vi "Destroy Session.vi"(8 "error in (no error)":errorcluster, 11 "Session Handle":refnum<data-value>) -> (0 "error out":errorcluster)   [LabVIEW 2020, in "G-Embedded-Python-Interpreter-Toolkit.lvlib"]
uses:
  G-Embedded-Python-Interpreter-Toolkit.lvlib
  bin/gepit.cp310.32.dll
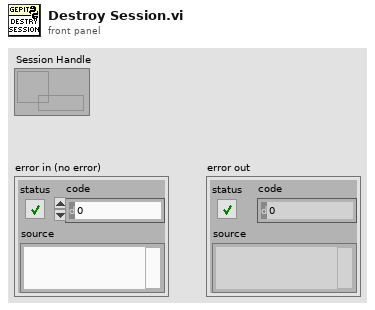
[diagram p1: front panel]
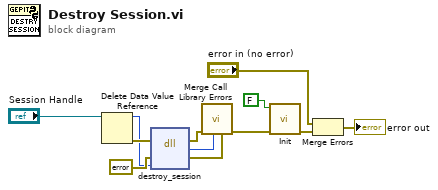
[diagram p0: block diagram]
diagram:
  n1 = Delete Data Value Reference(data value reference="Session Handle") -> (data value=w6:u64, error out=w7:errorcluster)  [unwired: 1 in]
  n2 = dll-call lib="C:/serenial/libraries/g-embedded-python-interpreter-toolkit/LabVIEW/bin/gepit.cp310.32.dll" fn="destroy_session"(error in=w7, "Error"=errorcluster {"status"=FALSE, "code"=0, "source"=""} ("error constant"), "Session"=w6) -> (error out=w11:errorcluster, "return type"=w10:i32, "Error"=w9:errorcluster)  [unwired: 3 in, 1 out]
  n3 = call "Merge Call Library Errors.vi"("Call Library Error"=w9, "Return Value"=w10, "error in"=w11) -> ("error out"=w3:errorcluster)  [unwired: 8 in]
  n4 = call "Init.vi"("error in (no error)"=w3, "Init"=FALSE) -> ("error out"=w2:errorcluster)  [unwired: 9 in]
  n5 = Merge Errors("error in (no error)", w2) -> (→"error out":errorcluster)
